vi "FireUpdateStatus.vi"(0 "object in":refnum<class "Application.lvclass">, 2 "Status":string, 5 "error in (no error)":errorcluster) -> (14 "object out":refnum<class "Application.lvclass">, 19 "error out":errorcluster)   [LabVIEW 2021, in "Application.lvclass"]
uses:
  Application.lvclass
  Application.lvclass/Application.ctl
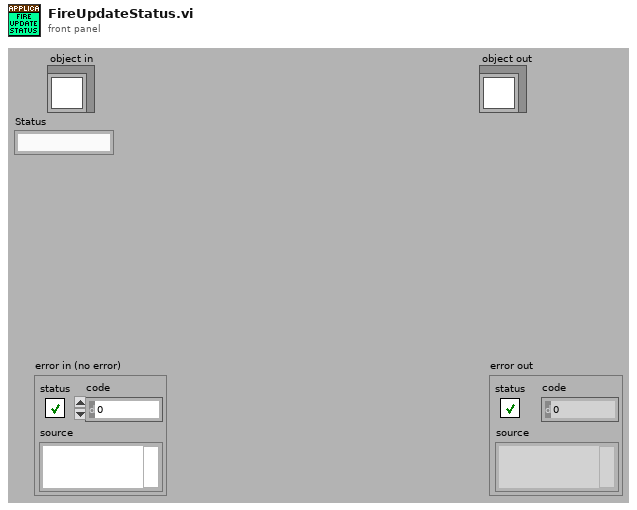
[diagram p1: front panel]
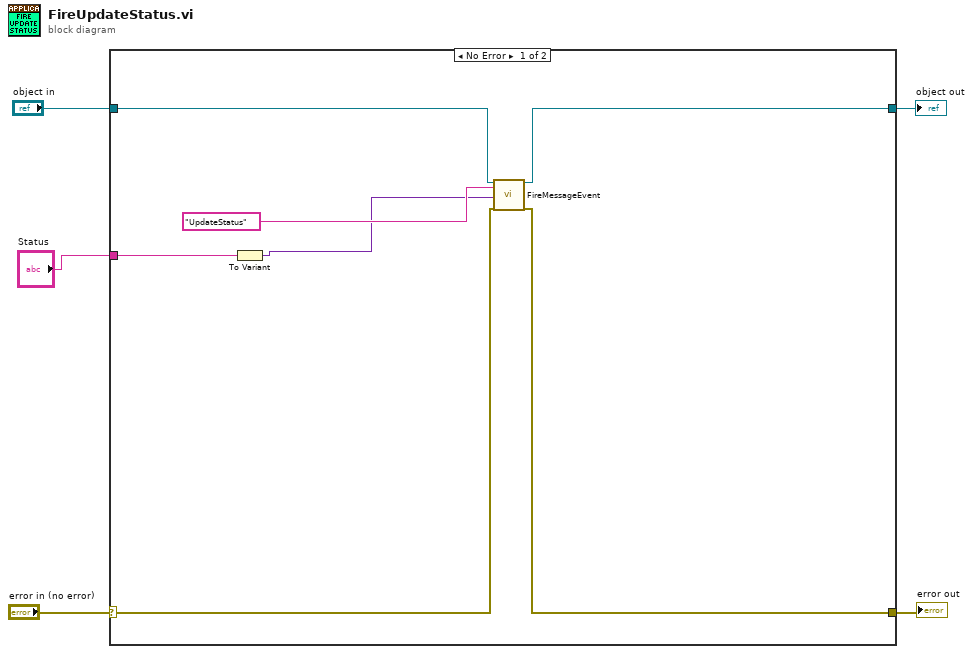
[diagram p0: block diagram]
diagram:
  n1 = case shown="No Error" "error in (no error)" {
    selector: "error in (no error)" -> [w9 w14]
    tunnel: [w8 w14] -> w4
    tunnel: [w11 w13] -> w2
    tunnel: "object in" -> [w10 w13]
    tunnel: "Status" -> [w12 _]
    frame No Error {
      n2 = To Variant(anything=w12) -> (Variant=w6:variant)
      n3 = call-dynamic "FireMessageEvent.vi"("object in"=w10, "Message"="UpdateStatus", "Message Data"=w6, "error in (no error)"=w9) -> ("object out"=w11:refnum<class "Application.lvclass">, "error out"=w8:errorcluster)  [unwired: 14 in]
    }
    frame Error {
    }
  }
  "error out" <- w4
  "object out" <- w2
